vi "Odd.vi"(7 "Odd":bool, 11 "Array In":dbl[][](array[numeric])) -> (3 "Array Out":dbl[][](array[numeric]))   [LabVIEW 2018]
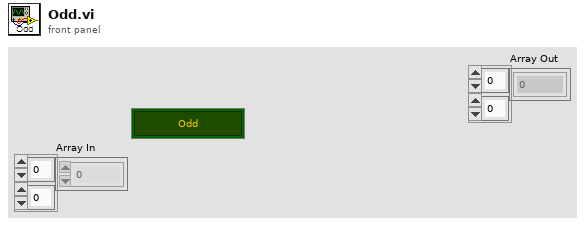
[diagram p1: front panel]
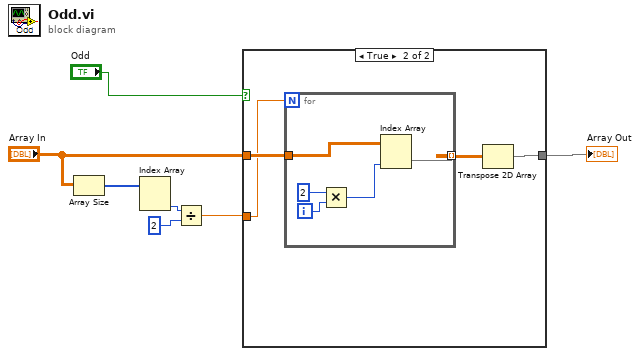
[diagram p0: block diagram]
diagram:
  n1 = Array Size(array="Array In") -> (size(s)=w6:i32[])
  n2 = Index Array(array=w6) -> (element #2=w3:i32)  [unwired: 2 in, 1 out]
  n3 = Divide(x=w3, y=2) -> (x/y=w4:dbl)
  n4 = case shown="True" "Odd" {
    tunnel: [w8 w9] -> w2
    tunnel: "Array In" -> [w8 w11]
    tunnel: w4 -> [_ w10]
    frame False {
    }
    frame True {
      n5 = for {
        N: w10 -> [_]
        tunnel: [w16] -> w12 mode=indexing
        tunnel: w11 -> [w17]
        i -> [w15]
        n6 = Multiply(x=2, y=w15) -> (x*y=w13:i32)
        n7 = Index Array(array=w17, index (col)=w13) -> (element=w16:dbl[])  [unwired: 1 in]
      }
      n8 = Transpose 2D Array(2D array=w12) -> (transposed array=w9:dbl[][])
    }
  }
  "Array Out" <- w2
